vi "Get Datagridview All Data.vi"(11 ".NET Refnum in":refnum<k24>) -> (1 "Row":i32, 2 ".NET Refnum in 2":refnum<k24>, 3 "Array":string[][](array[string]))   [LabVIEW 2013]
uses:
  System.Windows.Forms
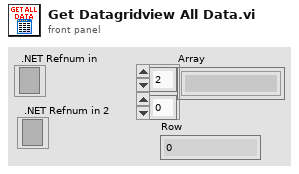
[diagram p1: front panel]
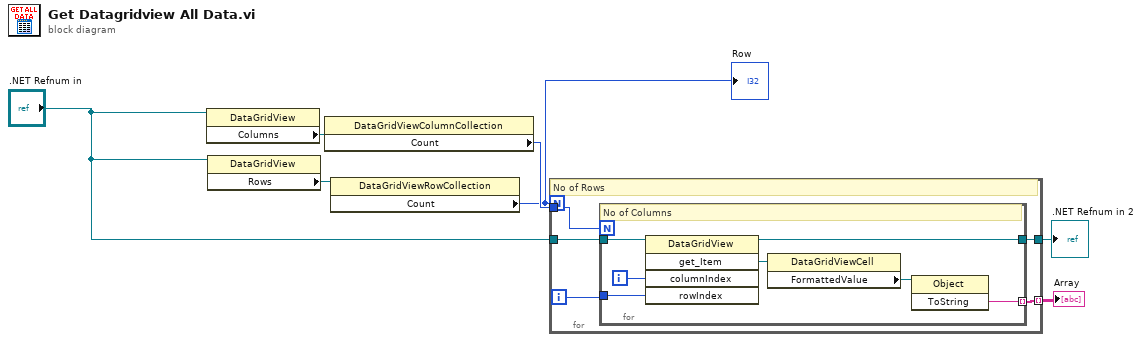
[diagram p0: block diagram]
diagram:
  n1 = property class="DataGridView"(reference=".NET Refnum in") -> ("Columns"=w3:refnum<k24>)  [unwired: 1 in, 2 out]
  n2 = property class="DataGridView"(reference=".NET Refnum in") -> ("Rows"=w2:refnum<k24>)  [unwired: 1 in, 2 out]
  n3 = property class="DataGridViewColumnCollection"(reference=w3) -> ("Count"=w5:i32)  [unwired: 1 in, 2 out]
  n4 = property class="DataGridViewRowCollection"(reference=w2) -> ("Count"=w4:i32)  [unwired: 1 in, 2 out]
  "Row" <- w4
  n5 = for {
    N: w4 -> [_]
    tunnel: w5 -> [w12]
    tunnel: ".NET Refnum in" -> [w11]
    tunnel: [w10] -> w7 mode=indexing
    tunnel: [w8] -> w1
    i -> [w9]
    # "No of Rows"
    n6 = for {
      N: w12 -> [_]
      tunnel: w11 -> [w18]
      tunnel: [w16] -> w10 mode=indexing
      tunnel: w9 -> [w14]
      tunnel: [w13] -> w8
      i -> [w17]
      # "No of Columns"
      n7 = invoke class="DataGridView" method="get_Item"(reference=w18, "columnIndex"=w17, "rowIndex"=w14) -> (reference out=w13:refnum<k24>, "get_Item"=w15:refnum<k24>)  [unwired: 2 in, 3 out]
      n8 = property class="DataGridViewCell"(reference=w15) -> ("FormattedValue"=w19:refnum<k24>)  [unwired: 1 in, 2 out]
      n9 = invoke class="Object" method="ToString"(reference=w19) -> ("ToString"=w16:string)  [unwired: 2 in, 2 out]
    }
  }
  "Array" <- w7
  ".NET Refnum in 2" <- w1
